vi "ElevatorGetPositionDemand.vi"() -> (7 "ShoulderPosDmdDeg":dbl)   [LabVIEW 2023]
doc: "Reads the Elevator's height demand from the Elevator Global ElevatorPosDemandHeight\n\nOutputs:\n--ElevHeight--numeric--inches"
uses:
  ElevatorGlobal.vi
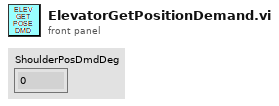
[diagram p1: front panel]
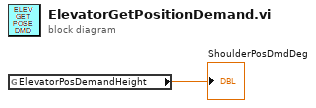
[diagram p0: block diagram]
diagram:
  n1 = global read "ElevatorGlobal.vi" "ElevatorPosDemandHeight"() -> (→"ShoulderPosDmdDeg":dbl)
